vi "Initialize.vi"(8 "error in (no error)":errorcluster, 11 "config file":path) -> (0 "error out":errorcluster, 3 "[User] Cfg File out":refnum<class "[User] Cfg File.lvclass">)   [LabVIEW 2020, in "[User] Cfg File.lvclass"]
uses:
  [User] Cfg File.lvclass
  [User] Cfg File.lvclass/[User] Cfg File.ctl
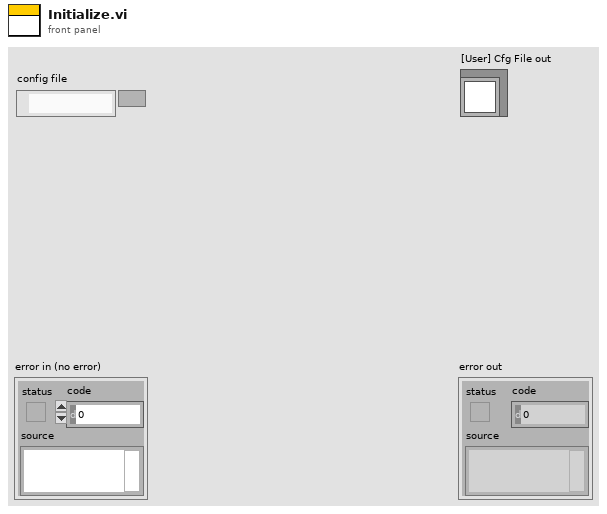
[diagram p1: front panel]
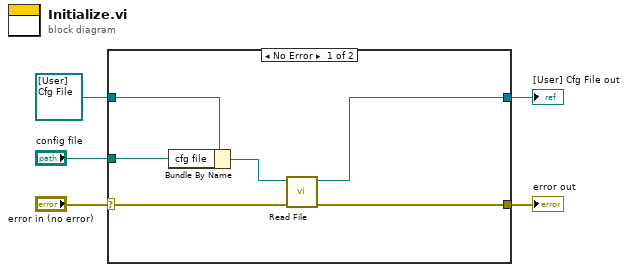
[diagram p0: block diagram]
diagram:
  n1 = case shown="No Error" "error in (no error)" {
    selector: "error in (no error)" -> [w9 w13]
    tunnel: [w7 w13] -> w4
    tunnel: [w6 w12] -> w2
    tunnel: refnum<class "[User] Cfg File.lvclass"> refnum ("[User] Cfg File in") -> [w11 w12]
    tunnel: "config file" -> [w10 _]
    frame No Error {
      n2 = Bundle By Name(cluster=w11, "cfg file"=w10) -> (w8:refnum<class "[User] Cfg File.lvclass">)
      n3 = call "Read File.vi"("error in (no error)"=w9, "[User] Cfg File in"=w8) -> ("error out"=w7:errorcluster, "[User] Cfg File out"=w6:refnum<class "[User] Cfg File.lvclass">)  [unwired: 8 in]
    }
    frame Error {
    }
  }
  "error out" <- w4
  "[User] Cfg File out" <- w2
